vi "PH_Sequencer.set i attribute.vi"(0 "i ref in":refnum<vi>, 2 "i attribute":T1={"GUI Refs"={"Main Off"=refnum, "Fire"=refnum, "Status"=refnum, "Ready"=refnum, "Waiting Time"=refnum, "Timeout"=refnum, "PPMA Ready"=refnum, "Sequencer SM State"=refnum, "PPPA Ready"=refnum, "Calorimeter"=refnum, "Beamline Ready"=refnum, "Clear Beamline"=refnum, "Linkage PPMA Rods"=refnum, "Linkage Current PA"=refnum, "Linkage Current MA"=refnum, "Timing Ready"=refnum, "State Timing"=refnum, "Force Timing"=refnum, "PSDB Shot Comment"=refnum, "State PA Backreflection"=refnum, "Beamline Z6 Ready"=refnum, "Clear Z6 Beamline"=refnum, "Sequence length"=refnum, "Timing Mode"=refnum, "Slow Trigger Settings"=refnum, "Experiment Description"=refnum, "State PSDB"=refnum, "PSDB Ready"=refnum, "Set PSDB Settings"=refnum, "Get PSDB Info"=refnum, "Take Snapshot"=refnum, "Shottype"=refnum, "Experiment"=refnum, "Phase Frontends"=refnum, "PP 45mm PILC in use"=refnum}, "Status Info"={"Machine Status"=0, "WaitingTime"=999969, "Timeout"=FALSE}, "Readyness"={"Ready to shot"=FALSE, "PPMA Ready"=FALSE, "PPPA Ready"=FALSE, "BL Ready"=FALSE, "Timing Ready"=FALSE, "BL Z6 Ready"=FALSE, "PSDBReady"=FALSE}, "Instancenames"={"PPMA Rods"="N/A", "PP Current Meas"="N/A", "PH Beamline Chief"="N/A", "PA Backrefl Meas"="N/A", "Z6 Beamline Chief"="N/A"}, "Data to read"=FALSE, "Calorimeter"={"Instancename"="N/A", "On"=FALSE, "linked"=FALSE}, "Linkage"={"PPMA Rods"=FALSE, "PP Current Meas"=FALSE, "PHELIX Beamline Chief"=FALSE, "PA Backrefl Meas"=FALSE, "Z6 Beamline Chief"=FALSE}, "Timing"={"Instance"="N/A", "linked"=FALSE, "Status"=0, "Timing Mode"={"T2"=0, "Modeselector"=enum."10 Hz"}, "Slow Trigger Settings"={"Delay"=0.0, "externally triggered?"=FALSE}, "Info available"={"ext SlowTrigger"=FALSE, "T2"=FALSE, "Mode"=FALSE, "Delay Slow Trigger"=FALSE, "Phase FEs"=FALSE}, "FE Phase"={"Phase"=0.0}}, "Service ID R2S"=-1, "PSDB"={"Controller Instance"="N/A", "Controller Status"=0, "Controller linked"=FALSE, "Settings acknowledged"=FALSE, "Current Experiment ID"=-1, "Current Shot Type"=-1, "Current Comment"="", "Remember Settings"=FALSE, "Write 2 early"=FALSE}, "PSDB Data"={"Main Off?"=FALSE, "Sequence Length"=0.0, "Sequence startet"=timestamp(0 s since 1904-01-01)}, "6P 4Q Positions"=[], "PUs"=[]} {"PUs"."Information"."State" items=["no info", "off/false/out", "on/true/in", "Failure", "Alarm", "Status 1", "Status 2", "Status 3"]; "6P 4Q Positions"."Position" items=["unknown", "Position I", "Position II", "Position III", "Position IV", "moving"]; "PSDB"."Controller Status" items=["no info", "off/false/out", "on/true/in", "Failure", "Alarm", "Status 1", "Status 2", "Status 3"]; "Timing"."FE Phase"."Phase" format="%#_12p"; "Timing"."Timing Mode"."T2" min=0 max=6000 step=2; "Timing"."Status" items=["no info", "off/false/out", "on/true/in", "Failure", "Alarm", "Status 1", "Status 2", "Status 3"]; "Status Info"."Machine Status" items=["no info", "off/false/out", "on/true/in", "Failure", "Alarm", "Status 1", "Status 2", "Status 3"]}, 5 "error in (no error)":errorcluster) -> (14 "i ref out":refnum<vi>, 19 "error out":errorcluster)   [LabVIEW 2014, in "PH_Sequencer.lvlib"]
doc: "Sets the i attribute data of an object.\n\nLicense Agreement for this software:\n\nCopyright (C)\nGesellschaft für Schwerionenforschung, GSI\nPlanckstr. 1\n64291 Darmstadt\nGermany\n\nContact: D.Beck@gsi.de \n\nThis program is free software; you can redistribute it and/or modify it under the terms of the GNU General Public License as published by the Free Software Foundation; either version 2 of the license, or (at your option) any later version.\n\nThis program is distributed in the hope that it will be useful, but WITHOUT ANY WARRANTY; without even the implied warranty of MERCHANTABILITY or FITNESS FOR A PARTICULAR PURPOSE. See the GNU General License for more details (http://www.gnu.org).\n\nGesellschaft für Schwerionenforschung, GSI\nPlanckstr. 1, 64291 Darmstadt, Germany\nFor all questions and ideas contact: M.Richter@gsi.de, H.Brand@gsi.de or D.Beck@gsi.de.\nLast update: 17-JUN-2004"
uses:
  PH_Sequencer.lvlib
  PH_Sequencer.i attribute.ctl
  PH_Basics/PH_StatusHandler/PH_StatusHandler.GUI element.ctl
  PH_Basics/PH_StatusHandler/PH_StatusHandler.Status.ctl
  PH_Timing/PH_Timing.Timing Mode.ctl
  PH_Timing/PH_Timing.Slow Trigger Settings.ctl
  PH_Timing/PH_Timing.Phase FEs.ctl
  PH_Motion/PH_4_Pos_Selector/PH_4_Pos_Selector.Position Selector.ctl
  PH_Sequencer.Head.ctl
  PH_Basics/PH_PP_Common/PH_PP_Common.PUs.ctl
  PH_Sequencer.PU Information for GUI.ctl
  PH_Basics/PH_PowerUnit_BaseClass/PH_PowerUnit_BaseClass.SM States.ctl
  PH_Sequencer.PU Information.ctl
  PH_Basics/PH_StatusHandler/PH_StatusHandler.lvlib
  PH_Timing/PH_Timing.lvlib
  PH_Motion/PH_4_Pos_Selector/PH_4_Pos_Selector.lvlib
  PH_Basics/PH_PP_Common/PH_PP_Common.lvlib
  PH_Basics/PH_PowerUnit_BaseClass/PH_PowerUnit_BaseClass.lvlib
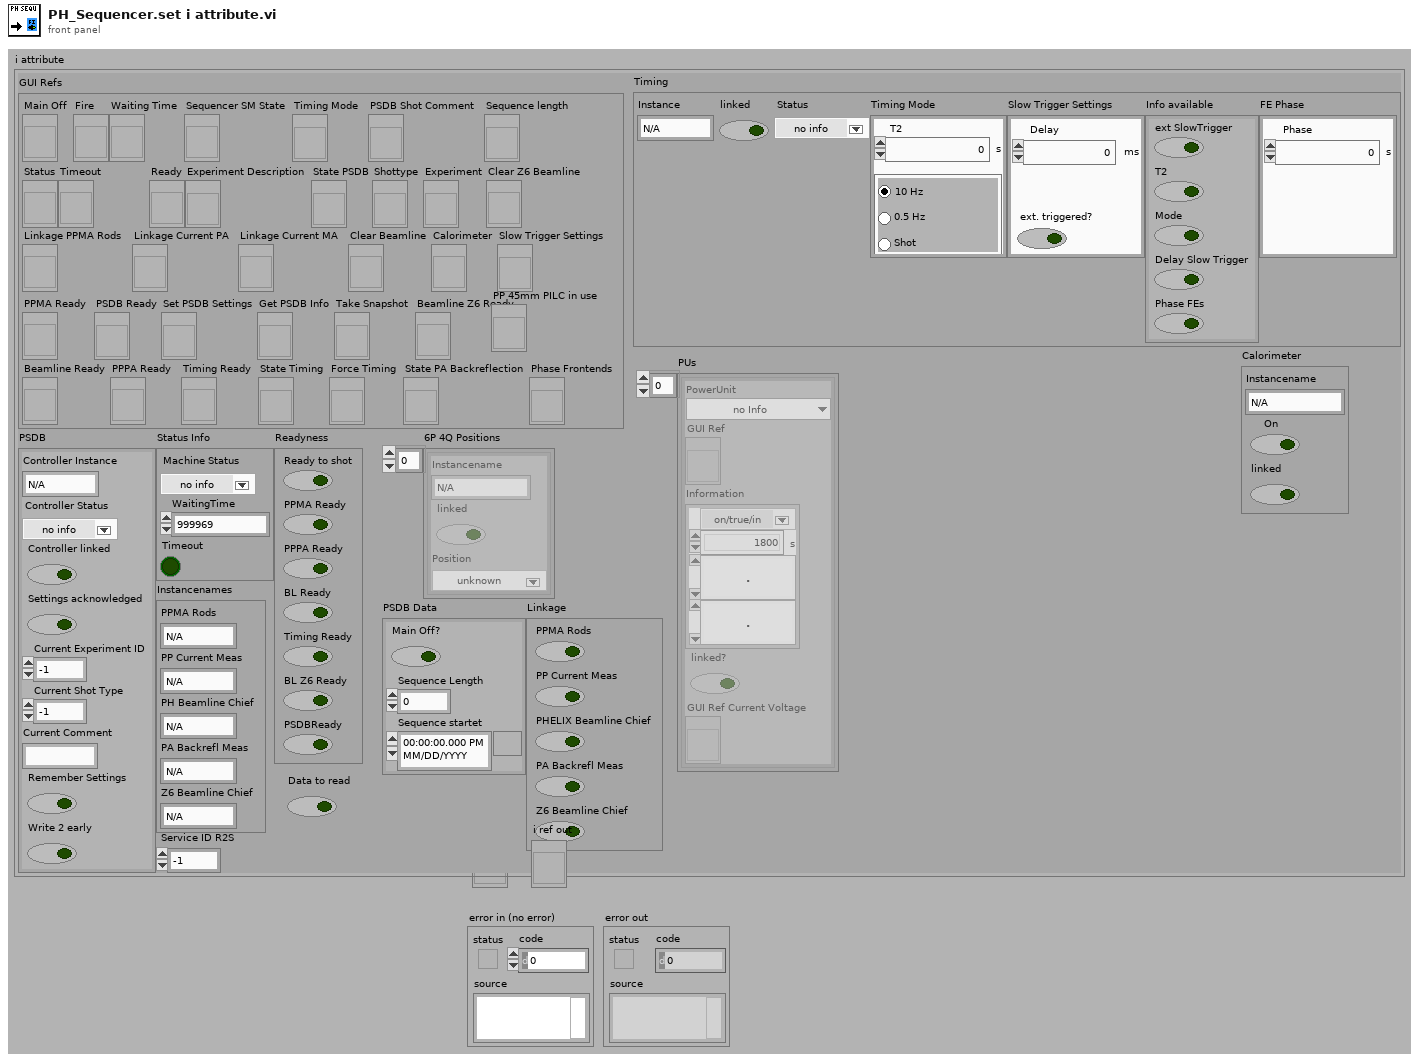
[diagram p1: front panel]
types:
  T1 = typedef "PH_Sequencer.lvlib/PH_Sequencer.i attribute.ctl" = cluster{"GUI Refs":cluster{"Main Off":refnum<vi>, "Fire":refnum<vi>, "Status":refnum<vi>, "Ready":refnum<vi>, "Waiting Time":refnum<vi>, "Timeout":refnum<vi>, "PPMA Ready":refnum<vi>, "Sequencer SM State":refnum<vi>, "PPPA Ready":refnum<vi>, "Calorimeter":refnum<vi>, "Beamline Ready":refnum<vi>, "Clear Beamline":refnum<vi>, "Linkage PPMA Rods":refnum<vi>, "Linkage Current PA":refnum<vi>, "Linkage Current MA":refnum<vi>, "Timing Ready":refnum<vi>, "State Timing":refnum<vi>, "Force Timing":refnum<vi>, "PSDB Shot Comment":refnum<vi>, "State PA Backreflection":refnum<vi>, "Beamline Z6 Ready":refnum<vi>, "Clear Z6 Beamline":refnum<vi>, "Sequence length":refnum<vi>, "Timing Mode":refnum<vi>, "Slow Trigger Settings":refnum<vi>, "Experiment Description":refnum<vi>, "State PSDB":refnum<vi>, "PSDB Ready":refnum<vi>, "Set PSDB Settings":refnum<vi>, "Get PSDB Info":refnum<vi>, "Take Snapshot":refnum<vi>, "Shottype":refnum<vi>, "Experiment":refnum<vi>, "Phase Frontends":refnum<vi>, "PP 45mm PILC in use":refnum<vi>}, "Status Info":cluster{"Machine Status":T2, "WaitingTime":i32, "Timeout":bool}, "Readyness":cluster{"Ready to shot":bool, "PPMA Ready":bool, "PPPA Ready":bool, "BL Ready":bool, "Timing Ready":bool, "BL Z6 Ready":bool, "PSDBReady":bool}, "Instancenames":cluster{"PPMA Rods":string, "PP Current Meas":string, "PH Beamline Chief":string, "PA Backrefl Meas":string, "Z6 Beamline Chief":string}, "Data to read":bool, "Calorimeter":cluster{"Instancename":string, "On":bool, "linked":bool}, "Linkage":cluster{"PPMA Rods":bool, "PP Current Meas":bool, "PHELIX Beamline Chief":bool, "PA Backrefl Meas":bool, "Z6 Beamline Chief":bool}, "Timing":cluster{"Instance":string, "linked":bool, "Status":T2, "Timing Mode":T3, "Slow Trigger Settings":T4, "Info available":cluster{"ext SlowTrigger":bool, "T2":bool, "Mode":bool, "Delay Slow Trigger":bool, "Phase FEs":bool}, "FE Phase":T5}, "Service ID R2S":i32, "PSDB":cluster{"Controller Instance":string, "Controller Status":T2, "Controller linked":bool, "Settings acknowledged":bool, "Current Experiment ID":i16, "Current Shot Type":i16, "Current Comment":string, "Remember Settings":bool, "Write 2 early":bool}, "PSDB Data":cluster{"Main Off?":bool, "Sequence Length":dbl, "Sequence startet":timestamp}, "6P 4Q Positions":cluster{"Instancename":string, "linked":bool, "Position":T6}[], "PUs":T7[]}
  T2 = typedef "PH_StatusHandler.lvlib/PH_StatusHandler.Status.ctl" = i16
  T3 = typedef "PH_Timing.lvlib/PH_Timing.Timing Mode.ctl" = cluster{"T2":i16, "Modeselector":enum32{"10 Hz", "0.5 Hz", "Shot"}}
  T4 = typedef "PH_Timing.lvlib/PH_Timing.Slow Trigger Settings.ctl" = cluster{"Delay":dbl, "externally triggered?":bool}
  T5 = typedef "PH_Timing.lvlib/PH_Timing.Phase FEs.ctl" = cluster{"Phase":dbl}
  T6 = typedef "PH_4_Pos_Selector.lvlib/PH_4_Pos_Selector.Position Selector.ctl" = u16
  T7 = typedef "PH_Sequencer.lvlib/PH_Sequencer.Head.ctl" = cluster{"PowerUnit":T8, "GUI Ref":refnum<vi>, "Information":T9, "linked?":bool, "GUI Ref Current Voltage":refnum<vi>}
  T8 = typedef "PH_PP_Common.lvlib/PH_PP_Common.PUs.ctl" = enum16{"no Info", "PA-19mm-1", "PA-19mm-2", "PA-45mm-PILC", "PA-45mm-MAIN", "MA-PU-1", "MA-PU-2", "MA-PU-3", "MA-PU-4", "MA-PU-5", "MA-PU-6", "MA-FR", "MA-PILC", "PA-45mm-DP"}
  T9 = typedef "PH_Sequencer.lvlib/PH_Sequencer.PU Information.ctl" = cluster{"State":T2, "Waiting Time [s]":dbl, "PU State SM":T10, "PU Timeout SM":T10}
  T10 = typedef "PH_PowerUnit_BaseClass.lvlib/PH_PowerUnit_BaseClass.SM States.ctl" = enum16{".", "Stand by", "Switch PU on", "Configure", "Set Default Voltage", "Set STANDBY", "Set READY", "Wait for Shot Cmd", "Open Dump Rods", "Open Ross Relais", "Close Ross Relais", "Switch PSU on", "Switch PSU off", "Charge", "Switch GD Channel on", "Close Dump Rods", "Rods-TO", "RR-TO", "PSU-TO", "Trigger-TO"}
  T11 = enum16{"SetAttribute", "GetAttribute", "CreateAttribute", "DestroyAttribute", "DestroyAllAtributes"}
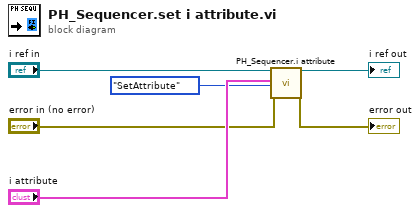
[diagram p0: block diagram]
diagram:
  n1 = call "PH_Sequencer.i attribute.vi"("VI Refnum"="i ref in", "CLASS.i attribute"="i attribute", "Action"=T11."SetAttribute", "error in (no error)"="error in (no error)") -> ("VI Refnum out"=→"i ref out":refnum<vi>, "error out"=→"error out":errorcluster)  [unwired: 13 in, 1 out]
